vi "Load Log Config from Preferences.vi"(8 "error in (no error)":errorcluster, 11 "User Preferences File in":refnum<class "User Preferences File.lvclass">) -> (0 "error out":errorcluster, 2 "Log Config":T1={"Log Level"=enum."WARNING"}, 3 "User Preferences File out":refnum<class "User Preferences File.lvclass">)   [LabVIEW 2020, in "RxnRover.lvlib"]
doc: "Updates the log configuration based on user preferences. This VI serves as a link between a User Preferences File object and the logging library without directly coupling the two.\n\nNOTE: The provided User Preferences object must already be initialized.\n\nTo view or update the log configuration at runtime, use the logging.lvlib:Set Log Config.vi and logging.lvlib:Get Log Config.vi VIs."
uses:
  RxnRover.lvlib
  User Preferences/User Preferences File.lvclass
  Log Config.ctl
  Log Levels.ctl
  logging.lvlib
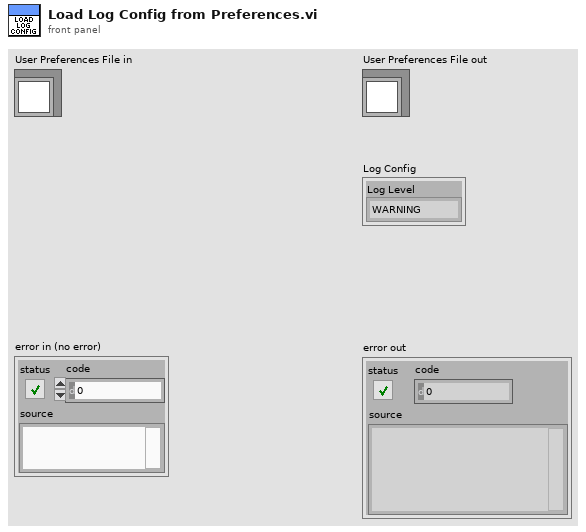
[diagram p1: front panel]
types:
  T1 = typedef "RxnRover.lvlib/logging.lvlib/Log Config.ctl" = cluster{"Log Level":T2}
  T2 = typedef "RxnRover.lvlib/logging.lvlib/Log Levels.ctl" = enum16{"NOTSET", "DEBUG", "INFO", "WARNING", "ERROR", "CRITICAL"}
  T3 = typedef "RxnRover.lvlib/User Preferences File.lvclass/User Preferences Cluster.ctl" = cluster{"Max Recent Experiments":dbl, "Recent Experiments":string[], "Log Level":string}
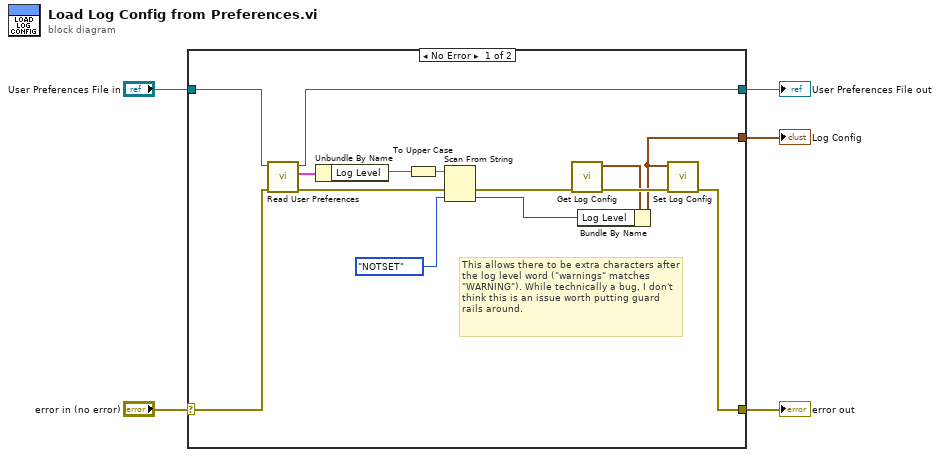
[diagram p0: block diagram]
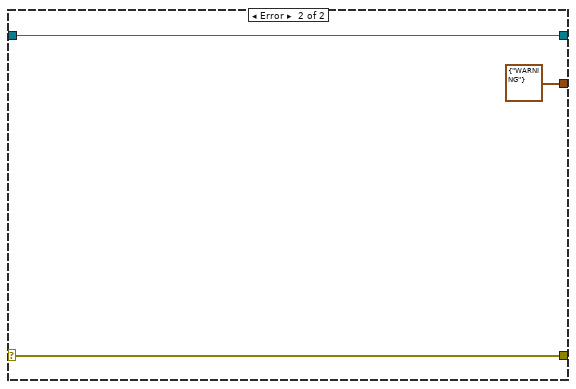
[diagram p2: hidden frame]
diagram:
  n1 = case shown="No Error" "error in (no error)" {
    selector: "error in (no error)" -> [w19 w22]
    tunnel: [w9 w22] -> w5
    tunnel: "User Preferences File in" -> [w17 w21]
    tunnel: [w18 w21] -> w2
    tunnel: [w6 T1 {"Log Level"=enum."WARNING"} ("Log Config")] -> w1
    frame No Error {
      # "This allows there to be extra characters after the log level word (\"warnings\" matches \"WARNING\"). While technically a bug, I don't think this is an issue worth putting guard rails around."
      n2 = call-dynamic "Read User Preferences.vi"("error in (no error)"=w19, "User Preferences File in"=w17) -> ("error out"=w11:errorcluster, "User Preferences"=w16:T3, "User Preferences File out"=w18:refnum<class "User Preferences File.lvclass">)  [unwired: 7 in]
      n3 = Unbundle By Name(w16) -> ("Log Level"=w7:string)
      n4 = To Upper Case(1:w7) -> (0:w8:string)
      n5 = Scan From String(input string=w8, error in=w11, default 1=Log_Levels."NOTSET" ("Log Level")) -> (error out=w10:errorcluster, output 1=w12:T2)  [unwired: 2 in, 2 out]
      n6 = call "Get Log Config.vi"("error in (no error)"=w10) -> ("error out"=w15:errorcluster, "Log Config"=w14:T1)  [unwired: 9 in]
      n7 = Bundle By Name(cluster=w14, "Log Level"=w12) -> (w6:T1)
      n8 = call "Set Log Config.vi"("error in (no error)"=w15, "Log Config"=w6) -> ("error out"=w9:errorcluster)  [unwired: 9 in]
    }
    frame Error {
    }
  }
  "error out" <- w5
  "User Preferences File out" <- w2
  "Log Config" <- w1
